vi "读取配置文件引用 i.vi"(8 "error in (no error)":errorcluster caption="错误输入（无错误）", 11 "段-输入":refnum<class "段-.lvclass">) -> (0 "error out":errorcluster caption="错误输出", 2 "配置文件引用":T1, 3 "段-输出":refnum<class "段-.lvclass">)   [LabVIEW 2017, in "项目开发助手.lvlib" / "模板-配置文件相关.lvlib" / "段-.lvclass"]
uses:
  <vilib>/Utility/config.llb/Config Data RefNum.ctl
  <vilib>/Utility/config.llb/NI_LVConfig.lvlib
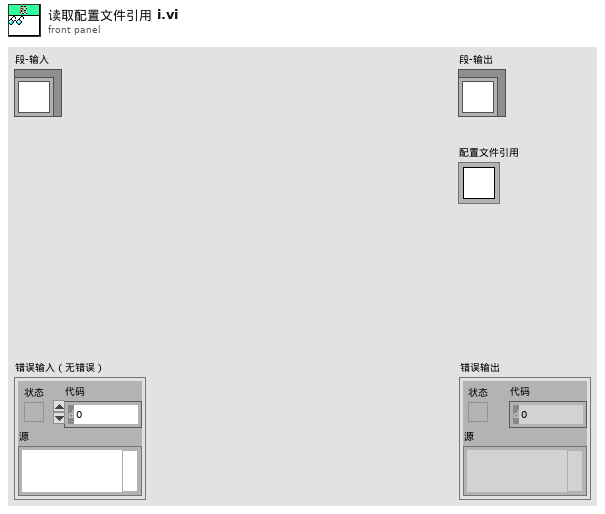
[diagram p1: front panel]
types:
  T1 = typedef "NI_LVConfig.lvlib/Config Data RefNum.ctl" = refnum<k1>
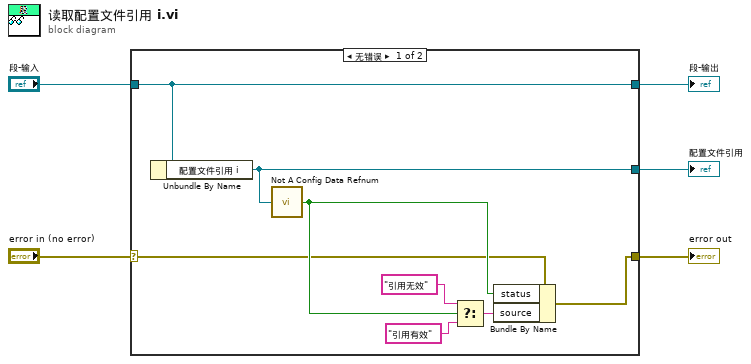
[diagram p0: block diagram]
diagram:
  n1 = case shown="无错误" "error in (no error)" {
    selector: "error in (no error)" -> [w7 w14]
    tunnel: [w6 w14] -> w4
    tunnel: [w13 w15] -> w2
    tunnel: "段-输入" -> [w13 w15]
    tunnel: [w9 _] -> w1
    frame No Error {
      n2 = Unbundle By Name(w13) -> ("配置文件引用 i"=w9:T1)
      n3 = call <vilib>:"Not A Config Data Refnum.vi"("refnum"=w9) -> ("not a config data refnum"=w8:bool)
      n4 = Select(t="引用无效", s=w8, f="引用有效") -> (s? t:f=w10:string)
      n5 = Bundle By Name(cluster=w7, "status"=w8, "source"=w10) -> (w6:errorcluster)
    }
    frame Error {
    }
  }
  "error out" <- w4
  "段-输出" <- w2
  "配置文件引用" <- w1
